vi "Device ID to Name.vi"(8 "Error In":errorcluster, 9 "Device ID":u8, 10 "Device Family":T1, 11 "LINX Device Config":T2) -> (0 "Error Out":errorcluster, 2 "Device Name":string, 3 "LINX Device Config":T2)   [LabVIEW 2018, in "LVH-LINX.lvlib"]
doc: "Get the device name from the device family and device ID."
uses:
  LVH-LINX.lvlib
  Device/Type Defs/LINX Device Config.ctl
  Type Defs/Interface.ctl
  Device/Type Defs/TCP Config.ctl
  Type Defs/Device Family.ctl
  Device/Device.lvlib
panel:
  out "Device ID":u8
  out "Device Family":T1
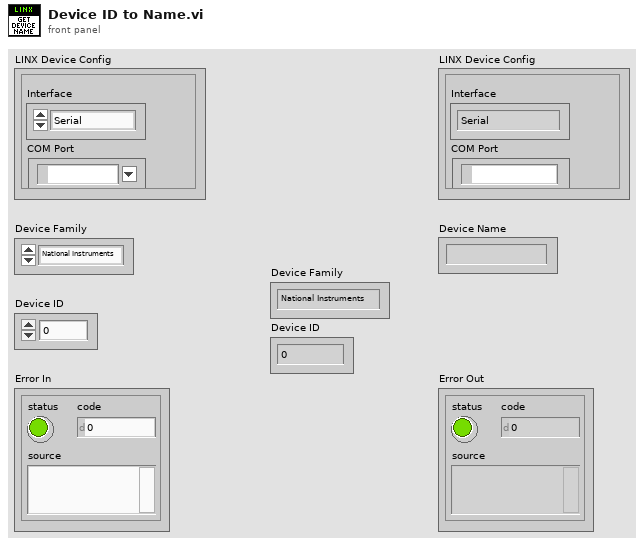
[diagram p1: front panel]
types:
  T1 = typedef "LVH-LINX.lvlib/Device Family.ctl" = enum8{"National Instruments", "Digilent", "Arduino"}
  T2 = typedef "LVH-LINX.lvlib/Device.lvlib/LINX Device Config.ctl" = cluster{"Interface":T3, "COM Port":refnum<visa-resource-name>, "TCP Configuration":T4, "Device Family":T1, "Device ID":u8, "Device Name":string, "TCP Ref":refnum<k5>}
  T3 = typedef "LVH-LINX.lvlib/Interface.ctl" = enum16{"Serial", "TCP"}
  T4 = typedef "LVH-LINX.lvlib/Device.lvlib/TCP Config.ctl" = cluster{"IP Address":string, "Port":u16}
  T5 = typedef "LVH-LINX.lvlib/Generic Device.ctl" = cluster{"DI Channels":u8[], "DO Channels":u8[], "AI":u8[], "AO":u8[], "PWM":u8[], "QE":u8[], "UART":u8[], "I2C 2":u8[], "SPI":u8[], "CAN":u8[], "AI Ref (V)":dbl, "Firmware Program Interfaces":enum16{"N/A", "Serial / USB", "USB", "TCP"}[], "Firmware Versions":T6[], "Name":string, "AO Resolution (Bits)":u8, "AO Ref (V)":dbl}
  T6 = typedef "LVH-LINX.lvlib/Firmware Version.ctl" = cluster{"Name":string, "Relative Path":string, "Firmware Interface":T7}
  T7 = typedef "LVH-LINX.lvlib/Firmware Interface.ctl" = enum32{"Serial ", "Ethernet", "WIFI"}
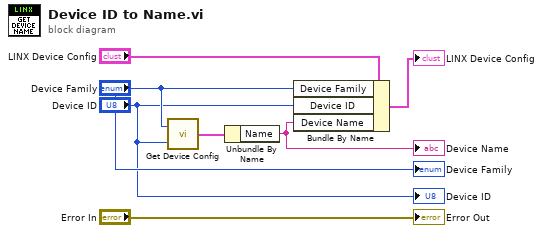
[diagram p0: block diagram]
diagram:
  n1 = call "Get Device Config.vi"("Device ID"="Device ID", "Device Family"="Device Family") -> ("Device Config"=w3:T5)
  n2 = Unbundle By Name(w3) -> ("Name"=w2:string)
  "Device Name" <- w2
  n3 = Bundle By Name(cluster="LINX Device Config", "Device Family"="Device Family", "Device ID"="Device ID", "Device Name"=w2) -> (→"LINX Device Config":T2)
  "Error Out" <- "Error In"
  "Device Family" <- "Device Family"
  "Device ID" <- "Device ID"
